vi "Reset Camera from file.vi"(8 "error in":errorcluster, 11 "Refnum in":T1) -> (0 "error out":errorcluster, 3 "Refnum out":T1)   [LabVIEW 2015, in "Camera SubVIs.lvlib"]
uses:
  Camera SubVIs.lvlib
  Calibration and Function folders.ctl
  <vilib>/userdefined/High Color/IMAQdx.ctl
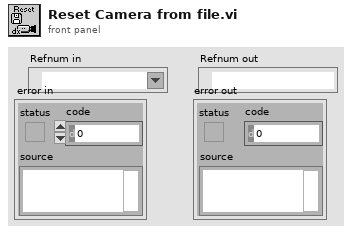
[diagram p1: front panel]
types:
  T1 = typedef "IMAQdx.ctl" = refnum<k21>
  T2 = typedef "Calibration and Function folders.ctl" = enum16{"Sensors", "Functions", "Config File", "PublicAppFolder", "New ini File", "Set Config File", "Delete ini File"}
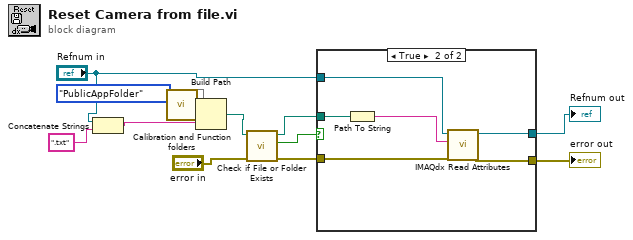
[diagram p0: block diagram]
diagram:
  n1 = Concatenate Strings("Refnum in", ".txt") -> (w3:string)
  n2 = call "Calibration and Function folders.vi"(11:Calibration_and_Function_folders."PublicAppFolder" ("Folder")) -> (7:w1)  [unwired: 8 in, 2 out]
  n3 = Build Path(base path=w1, name or relative path=w3) -> (appended path=w9:path)
  n4 = call <vilib>:"Check if File or Folder Exists.vi"("error in (no error)"="error in", "path"=w9) -> ("error out"=w7:errorcluster, "file or folder exists?"=w6:bool, "dup path"=w8:path)  [unwired: 7 in]
  n5 = case shown="True" w6 {
    tunnel: [w13 w20] -> w12
    tunnel: w8 -> [_ w18]
    tunnel: [w14 w17] -> w11
    tunnel: "Refnum in" -> [w13 w16]
    tunnel: w7 -> [w14 w15]
    frame False {
    }
    frame True {
      n6 = Path To String(path=w18) -> (string=w19:string)
      n7 = call <vilib>:"IMAQdx Read Attributes.vi"("error in"=w15, "Filename"=w19, "Session In"=w16) -> ("error out"=w17:errorcluster, "Session Out"=w20:T1)  [unwired: 7 in]
    }
  }
  "Refnum out" <- w12
  "error out" <- w11
